vi "DDSSequence_Build.vi"(6 "Freqeuncy (MHz)":dbl[][](array[numeric]), 7 "Power":dbl[][](array[numeric]), 9 "Channels":T1(ring), 10 "Duration (ms)":dbl[][](array[numeric]), 11 "No of  active time blocks":dbl) -> (3 "appended instruction string":string)   [LabVIEW 2016]
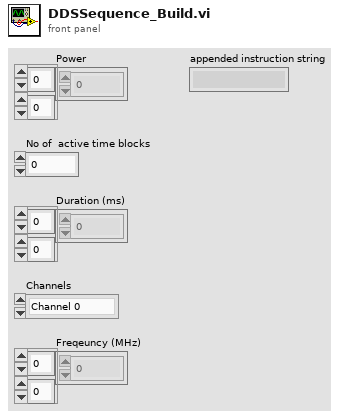
[diagram p1: front panel]
types:
  T1 = enum32{"Channel 0", "Channel 1", "Both channels"}
  T2 = enum32{"O_RAMP_SWP_OVR", "RAM_SWP_OVR", "O_DROVER", "DROVER", "O_SPI_FIFO_EV1", "SPI_FIFO_EV1", "O_SPI_FIFO_EV0", "SPI_FIFO_EV0", "O_SPI_FIFO_FLUSHED", "SPI_FIFO_FLUSHED", "BNC_IN_B_LEVEL", "BNC_IN_B_FALLING", "BNC_IN_B_RISING", "BNC_IN_A_LEVEL", "BNC_IN_A_FALLING", "BNC_IN_A_RISING", "ALL_SPI_FIFOS_FLUSHED", "NONE"}
  T3 = cluster{"Enable ASF from STP (F)":bool, "Digital ramp enable (F)":bool, "Digital ramp no-dwell high (F)":bool, "Digital ramp no-dwell low (F)":bool, "Matched latency enable (T)":bool, "Parallel data port enable (F)":bool}
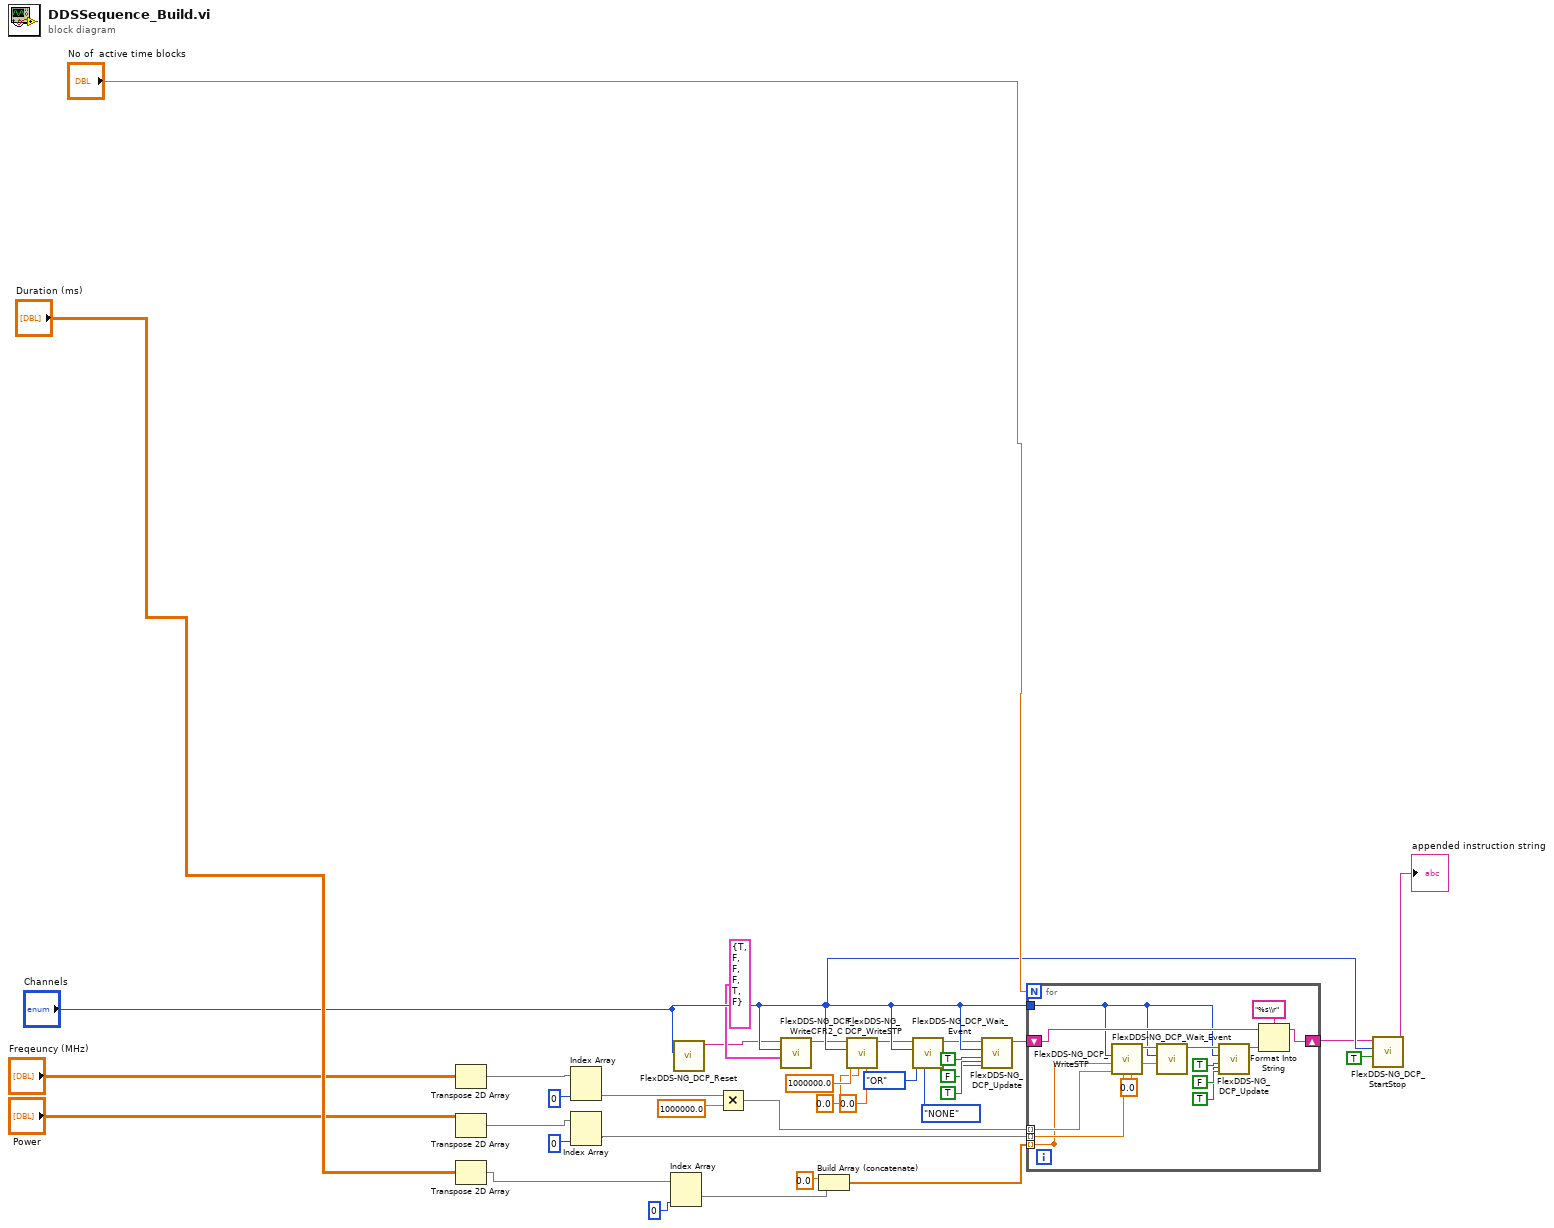
[diagram p0: block diagram]
diagram:
  n1 = Transpose 2D Array(2D array="Freqeuncy (MHz)") -> (transposed array=w26:dbl[][])
  n2 = Transpose 2D Array(2D array="Power") -> (transposed array=w23:dbl[][])
  n3 = Transpose 2D Array(2D array="Duration (ms)") -> (transposed array=w35:dbl[][])
  n4 = Index Array(array=w26, index (col)=0 ("index (row)")) -> (element=w28:dbl[])  [unwired: 1 in]
  n5 = Index Array(array=w23, index (col)=0 ("index (row)")) -> (element=w24:dbl[])  [unwired: 1 in]
  n6 = Index Array(array=w35, index (col)=0 ("index (row)")) -> (element=w32:dbl[])  [unwired: 1 in]
  n7 = call "FlexDDS-NG_DCP_Reset.vi"("Channels"="Channels") -> ("appended instruction string"=w2:string)  [unwired: 10 in]
  n8 = Multiply(x=w28, y=1000000.0 ("frequency Hz (0..400M)")) -> (x*y=w20:dbl[])
  n9 = call "FlexDDS-NG_DCP_WriteCFR2_C.vi"("CFR2 bits"=T3 {"Enable ASF from STP (F)"=TRUE, "Digital ramp enable (F)"=FALSE, "Digital ramp no-dwell high (F)"=FALSE, "Digital ramp no-dwell low (F)"=FALSE, "Matched latency enable (T)"=TRUE, "Parallel data port enable (F)"=FALSE} ("CFR2 bits 2"), "Channels"="Channels", "initial instruction string"=w2) -> ("appended instruction string"=w6:string)  [unwired: 8 in]
  n10 = Build Array (concatenate)(0.0 ("phase degrees (0..360)"), w32) -> (w33:dbl[])
  n11 = call "FlexDDS-NG_DCP_WriteSTP.vi"("phase degrees (0..360)"=0.0, "amplitude (0..1)"=0.0, "frequency Hz (0..400M)"=1000000.0, "Channels"="Channels", "initial instruction string"=w6) -> ("appended instruction string"=w11:string)  [unwired: 6 in]
  n12 = call "FlexDDS-NG_DCP_Wait_Event.vi"("Event 1"=T2."NONE", "AND/OR"=enum32{"AND", "OR"}."OR", "Channels in"="Channels", "appended instruction string in"=w11) -> ("appended instruction string"=w10:string)  [unwired: 7 in]
  n13 = call "FlexDDS-NG_DCP_Update.vi"("ONLY IO_UPDATE"=TRUE, "DRCTL(true=+, false=-)"=FALSE ("DRCTL(true=+, false=-) 2"), "IO_UPDATE(true=u, false = '')"=TRUE ("IO_UPDATE(true=u, false = '')  2"), "Channels"="Channels", "appended instruction string in"=w10) -> ("appended instruction string out"=w16:string)  [unwired: 6 in]
  n14 = for {
    N: "No of  active time blocks" -> [_]
    shift-right: [w41] -> w17
    shift-left: w16 -> [w42]
    tunnel: w24 -> [w39] mode=indexing
    tunnel: "Channels" -> [w38]
    tunnel: w33 -> [w36] mode=indexing
    tunnel: w20 -> [w37] mode=indexing
    tunnel: [w36] -> _ mode=indexing
    n15 = call "FlexDDS-NG_DCP_WriteSTP.vi"("phase degrees (0..360)"=0.0, "amplitude (0..1)"=w39, "frequency Hz (0..400M)"=w37, "Channels"=w38) -> ("appended instruction string"=w44:string)  [unwired: 7 in]
    n16 = call "FlexDDS-NG_DCP_Wait_Event.vi"("waiting time [ms]"=w36, "Channels in"=w38, "appended instruction string in"=w44) -> ("appended instruction string"=w45:string)  [unwired: 8 in]
    n17 = call "FlexDDS-NG_DCP_Update.vi"("ONLY IO_UPDATE"=TRUE, "DRCTL(true=+, false=-)"=FALSE ("DRCTL(true=+, false=-) 2"), "IO_UPDATE(true=u, false = '')"=TRUE ("IO_UPDATE(true=u, false = '')  2"), "Channels"=w38, "appended instruction string in"=w45) -> ("appended instruction string out"=w40:string)  [unwired: 6 in]
    n18 = Format Into String(format string="%s\\r", initial string=w42, w40) -> (resulting string=w41:string)  [unwired: 1 in, 1 out]
  }
  n19 = call "FlexDDS-NG_DCP_StartStop.vi"("start (T) stop (F)"=TRUE, "Channels"="Channels", "initial instruction string"=w17) -> ("appended instruction string"=→"appended instruction string":string)  [unwired: 8 in]
